vi "test6.4-RegisterInterruptAsStatusFromNonCSM.vi"(8 "error in (no error)":errorcluster, 11 "TestCase in":refnum<class "testcase-CSMBroadcast.lvclass">) -> (0 "error out":errorcluster, 3 "TestCase out":refnum<class "testcase-CSMBroadcast.lvclass">)   [LabVIEW 2017, in "testcase-CSMBroadcast.lvclass"]
uses:
  testcase-CSMBroadcast.lvclass
  src/user.lib/_NEVSTOP/Communicable State Machine(CSM)/AdvanceAPI/CSM - Broadcast Message Type.ctl
  <vilib>/addons/_JKI Toolkits/VI Tester/TestCase.llb/TestCase.lvclass
  src/user.lib/_NEVSTOP/Communicable State Machine(CSM)/Communicable State Machine.lvlib
  C:/Program Files (x86)/National Instruments/LabVIEW 2017/vi.lib/addons/_JKI Toolkits/VI Tester/TestCase.llb/TestCase.lvclass
panel:
  out "output cluster":T1
  out "error out 3":errorcluster
  out "error out 2":errorcluster
  out "LoopCount":i32
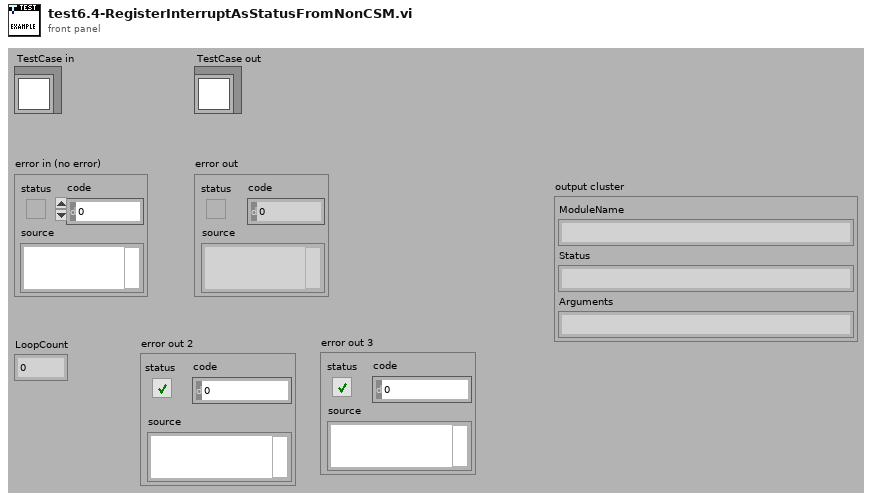
[diagram p1: front panel]
types:
  T1 = cluster{"ModuleName":string, "Status":string, "Arguments":string}
  T2 = typedef "Communicable State Machine.lvlib/CSM - Broadcast Message Type.ctl" = enum16{"<Null>", "Status", "Interrupt"}
  T3 = cluster{"Status Event":refnum<user-event>, "Interrupt Event":refnum<user-event>}
  T4 = cluster{"cluster":cluster{"ModuleName":string, "Status":string, "Arguments":string}}
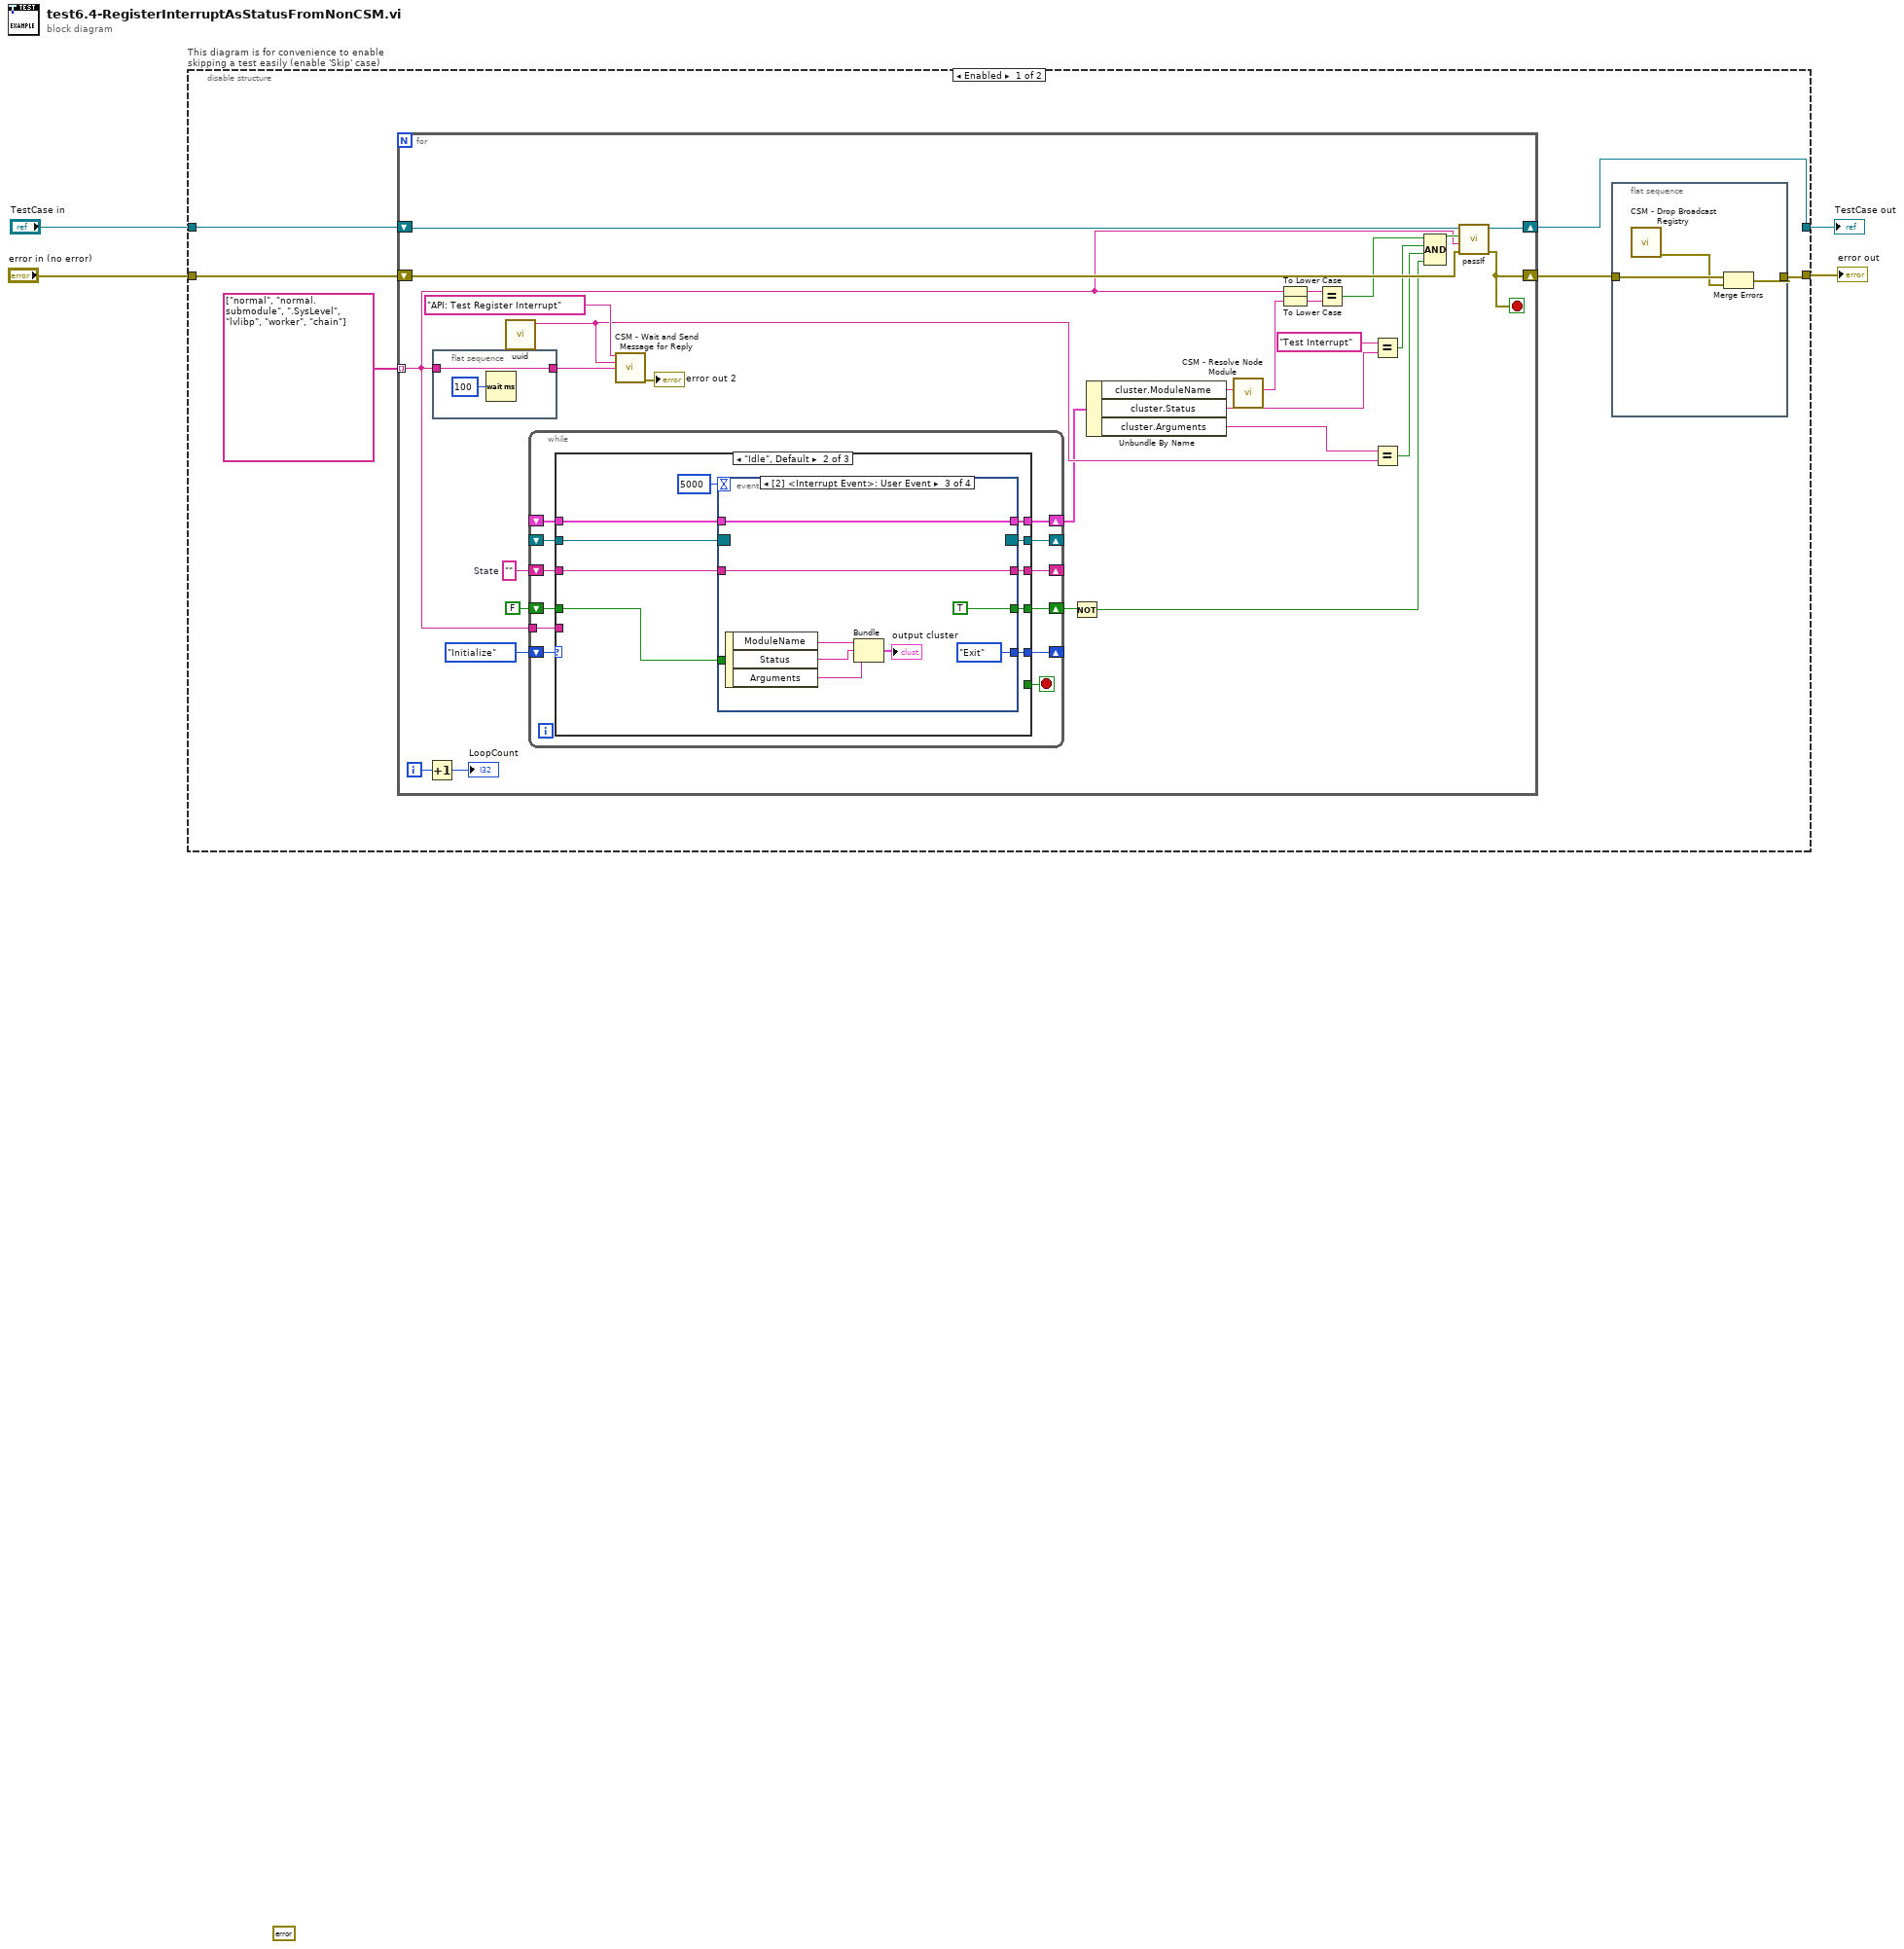
[diagram p0: block diagram]
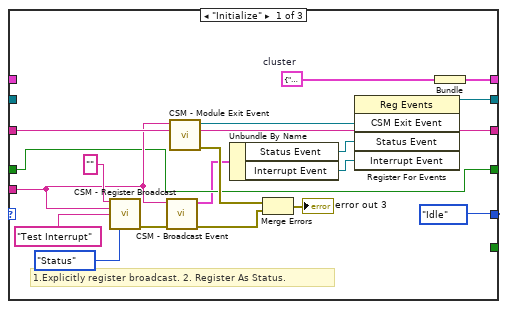
[diagram p2: hidden frame]
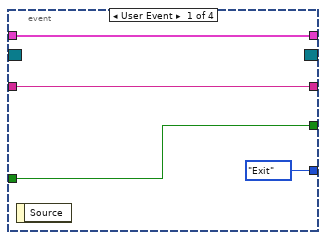
[diagram p3: hidden frame]
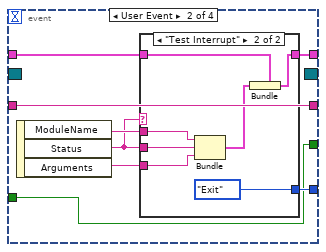
[diagram p4: hidden frame]
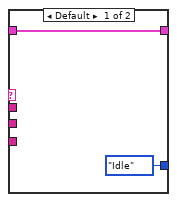
[diagram p5: hidden frame]
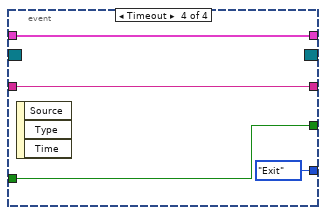
[diagram p6: hidden frame]
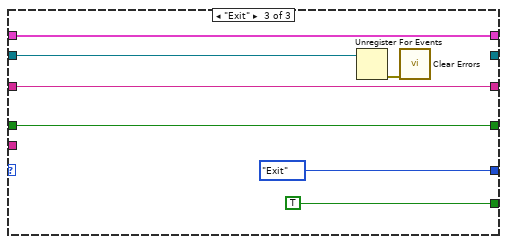
[diagram p7: hidden frame]
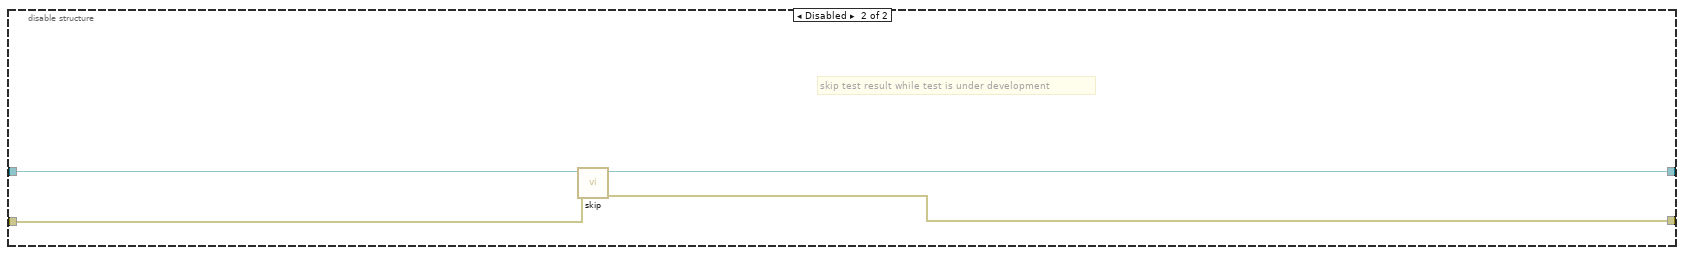
[diagram p8: hidden frame]
diagram:
  (unwired) errorcluster {"status"=FALSE, "code"=0, "source"=""} ("error out")
  n1 = disable-structure "This diagram is for convenience to enable skipping a test easily (enable 'Skip' case)" shown="Enabled" {
    disable-tunnel: "TestCase in" -> [w10 w127]
    disable-tunnel: [w6 w125] -> w2
    disable-tunnel: [w5 w126] -> w1
    disable-tunnel: "error in (no error)" -> [w9 w124]
    frame Enabled {
      n2 = for {
        shift-right: [w32] -> w6
        shift-left: w10 -> [w33]
        tunnel: string[] ["normal", "normal.submodule", ".SysLevel", "lvlibp", "worker", "chain"] -> [w18] mode=indexing
        shift-right: [w23] -> w7
        shift-left: w9 -> [w31]
        i -> [w26]
        stop <- w23 stop-if-true
        w40 = ""  # State
        n3 = Increment(x=w26) -> (x+1=→"LoopCount":i32)
        n4 = flat-sequence {
          tunnel: w18 -> [w43]
          tunnel: [w43] -> w38
          frame #0 {
            n5 = Wait (ms)(milliseconds to wait=u32 100) -> ()  [unwired: 1 out]
          }
        }
        n6 = call "uuid.vi"() -> ("UUID"=w35:string)  [unwired: 11 in]
        n7 = while {
          shift-right: [w54] -> _
          shift-left: enum16{"Idle", "Initialize", "Exit"}."Initialize" -> [w55]
          shift-right: [w51] -> _
          shift-left: w40 -> [w52]
          shift-right: [w50] -> _
          shift-left: _ -> [w49]
          shift-right: [w48] -> w22
          shift-left: _ -> [w47]
          tunnel: w18 -> [w46]
          shift-right: [w45] -> w16
          shift-left: FALSE -> [w44]
          stop <- w53 stop-if-true
          n8 = case shown="\"Idle\", Default" w55 {
            tunnel: [enum16{"Idle", "Initialize", "Exit"}."Idle" w83 enum16{"Idle", "Initialize", "Exit"}."Exit"] -> w54
            tunnel: [_ _ TRUE] -> w53
            tunnel: w52 -> [w72 w81 w121]
            tunnel: [w72 w82 w121] -> w51
            tunnel: [w70 w79 _] -> w50
            tunnel: w49 -> [_ w80 w120]
            tunnel: [w69 w77 w118] -> w48
            tunnel: w47 -> [_ w78 w118]
            tunnel: w46 -> [w61 _ _]
            tunnel: [w58 w75 w117] -> w45
            tunnel: w44 -> [w58 w74 w117]
            frame "Initialize" {
              w68 = T1 {"ModuleName"="", "Status"="", "Arguments"=""}  # cluster
              # "1.Explicitly register broadcast. 2. Register As Status."
              n9 = call "CSM - Register Broadcast.vi"("CSM Name(Empty for Broadcast Event)"="", "Source CSM Name (* as Default)"=w61, "Trigger"="Test Interrupt" ("State"), "Priority(No Change)"=CSM_-_Broadcast_Message_Type."Status") -> ("error out"=w63:errorcluster)  [unwired: 10 in, 1 out]
              n10 = call "CSM - Broadcast Event.vi"("Error In"=w63, "CSM Module"=w61) -> ("error out"=w66:errorcluster, "Broadcast Event"=w57:T3)  [unwired: 7 in, 1 out]
              n11 = call "CSM - Module Exit Event.vi"("Name (\"\" to Use UUID) In"=w61) -> ("error out"=w67:errorcluster, "CSM Exit Event"=w71:refnum<user-event>)  [unwired: 8 in, 1 out]
              n12 = Unbundle By Name(w57) -> ("Status Event"=w60:refnum<user-event>, "Interrupt Event"=w59:refnum<user-event>)
              n13 = Merge Errors(w67, w66) -> (→"error out 3":errorcluster)
              n14 = register-events(w71, w60, w59) -> (reference out=w70:refnum<event-registration>)  [unwired: 2 in, 1 out]
              n15 = Bundle("cluster"=w68) -> (w69:T4)  [unwired: 1 in]
            }
            frame "Idle", Default {
              n16 = event shown="[2] <Interrupt Event>: User Event" {
                selector: w80 -> [_ _ _ _]
                dyn-events: [_ _ _ _] -> w79
                timeout: 5000 -> [_ _ _ _]
                tunnel: [enum16{"Idle", "Initialize", "Exit"}."Exit" w94 enum16{"Idle", "Initialize", "Exit"}."Exit" enum16{"Idle", "Initialize", "Exit"}."Exit"] -> w83
                tunnel: w81 -> [w87 w95 w112 w116]
                tunnel: [w87 w95 w112 w116] -> w82
                tunnel: w78 -> [w85 w91 w111 w115]
                tunnel: [w85 w90 w111 w115] -> w77
                tunnel: [w84 w88 TRUE w113] -> w75
                tunnel: w74 -> [w84 w88 _ w113]
                event User Event {
                  n17 = event-data() -> ()  [unwired: 1 in, 1 out]
                }
                event User Event {
                  n18 = event-data() -> ("ModuleName"=w93:string, "Status"=w89:string, "Arguments"=w92:string)  [unwired: 1 in]
                  n19 = case shown="\"Test Interrupt\"" w89 {
                    tunnel: [enum16{"Idle", "Initialize", "Exit"}."Idle" enum16{"Idle", "Initialize", "Exit"}."Exit"] -> w94
                    tunnel: w93 -> [_ w103]
                    tunnel: w89 -> [_ w102]
                    tunnel: w92 -> [_ w101]
                    tunnel: w91 -> [w97 w100]
                    tunnel: [w97 w98] -> w90
                    frame Default {
                    }
                    frame "Test Interrupt" {
                      n20 = Bundle("ModuleName"=w103, "Status"=w102, "Arguments"=w101) -> (w99:T1)  [unwired: 1 in]
                      n21 = Bundle(cluster=w100, "cluster"=w99) -> (w98:T4)
                    }
                  }
                }
                event User Event {
                  n22 = event-data() -> ("ModuleName"=w108:string, "Status"=w107:string, "Arguments"=w106:string)  [unwired: 1 in]
                  n23 = Bundle("ModuleName"=w108, "Status"=w107, "Arguments"=w106) -> (→"output cluster":T1)  [unwired: 1 in]
                }
                event Timeout {
                  n24 = event-data() -> ()  [unwired: 1 in, 3 out]
                }
              }
            }
            frame "Exit" {
              n25 = Unregister For Events(event registration refnum=w120) -> (error out=w119:errorcluster)  [unwired: 1 in]
              n26 = call <vilib>:"Clear Errors.vi"("error in (no error)"=w119) -> ()  [unwired: 5 in, 2 out]
            }
          }
        }
        n27 = call "CSM - Wait and Send Message for Reply.vi"("State"="API: Test Register Interrupt", "Arguments (\"\")"=w35, "Target Module"=w38) -> ("error out"=→"error out 2":errorcluster)  [unwired: 10 in, 2 out]
        n28 = Not(x=w16) -> (.not. x?=w15:bool)
        n29 = Unbundle By Name(w22) -> ("cluster.ModuleName"=w20:string, "cluster.Status"=w36:string, "cluster.Arguments"=w34:string)
        n30 = call "CSM - Resolve Node Module.vi"("Node Name"=w20) -> ("CSM Module Name"=w17:string)  [unwired: 10 in]
        n31 = To Lower Case(string=w18) -> (all lower case string=w21:string)
        n32 = To Lower Case(string=w17) -> (all lower case string=w19:string)
        n33 = Equal?(x=w21, y=w19) -> (x = y?=w30:bool)
        n34 = Equal?(x="Test Interrupt" ("State"), y=w36) -> (x = y?=w29:bool)
        n35 = Equal?(x=w34, y=w35) -> (x = y?=w28:bool)
        n36 = Compound Arithmetic op=AND(w30, w29, w28, w15) -> (w27:bool)
        n37 = call-dynamic "passIf.vi"("error in (no error)"=w31, "message (\"\")"=w18, "pass"=w27, "TestCase in"=w33) -> ("error out"=w23:errorcluster, "TestCase out"=w32:refnum<class "testcase-CSMBroadcast.lvclass">)  [unwired: 6 in]
      }
      n38 = flat-sequence {
        tunnel: w7 -> [w13]
        tunnel: [w12] -> w5
        frame #0 {
          n39 = call "CSM - Drop Broadcast Registry.vi"() -> ("error out"=w11:errorcluster)  [unwired: 15 in]
          n40 = Merge Errors(w13, w11) -> (w12:errorcluster)
        }
      }
    }
    frame Disabled {
      # "skip test result while test is under development"
      n41 = call <vilib>:"skip.vi"("error in (no error)"=w124, "TestCase in"=w127) -> ("error out"=w126:errorcluster, "TestCase out"=w125:refnum<class "testcase-CSMBroadcast.lvclass">)  [unwired: 8 in]
    }
  }
  "error out" <- w1
  "TestCase out" <- w2
